vi "Sensor Simulation RT Driver VI.vi"(7 "Operation":T1, 11 "Device Reference in":T2 format="%.0x") -> (0 "Error Code":i32)   [LabVIEW 2011, in "Sensor Simulation Custom Device.lvlib"]
uses:
  Sensor Simulation Custom Device.lvlib
  <vilib>/NI Veristand/Custom Device API/Custom Device Item Ref.ctl
  <vilib>/NI Veristand/Custom Device API/Hardware Interface Driver VI Operation.ctl
  TypeDefs/SensorStateVariables.ctl
  TypeDefs/4 Wire xVDT Parameters.ctl
  TypeDefs/5 Wire xVDT Parameters.ctl
  TypeDefs/Resolver Parameters.ctl
  <userlib>/_FPGA Interface Advanced Tools/FPGA Interface Base/FPGA Interface Base.lvclass
  <vilib>/NI Veristand/Custom Device API/Block Data Reference.ctl
  <vilib>/NI Veristand/Custom Device API/Data Reference.ctl
  <vilib>/NI Veristand/Custom Device API/Data Access Type.ctl
  <vilib>/NI Veristand/Custom Device API/Custom Device Channel Type.ctl
  <userlib>/_FPGA Interface Advanced Tools/FPGA Interface Wrapper/NiFPGA Write.vi
  <userlib>/_FPGA Interface Advanced Tools/FPGA Interface Wrapper/NiFPGA Write - I32.vi
  <vilib>/NI Veristand/Custom Device API/NI VeriStand - Get Channel Values by Block Data Reference.vi
  <userlib>/_FPGA Interface Advanced Tools/FPGA Interface Base/Accessors/FPGA Read Session.vi
  <vilib>/NI Veristand/Custom Device API/Global Data Refs.vi
  <vilib>/Utility/error.llb/Error Cluster From Error Code.vi
  <vilib>/NI Veristand/Custom Device API/Custom Device API.lvlib
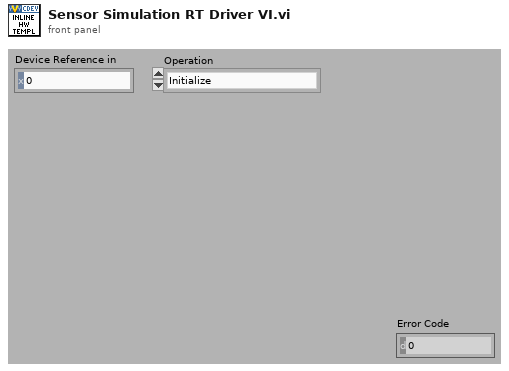
[diagram p1: front panel]
types:
  T1 = typedef "Custom Device API.lvlib/Hardware Interface Driver VI Operation.ctl" = enum16{"Initialize", "Start", "Read Data from HW", "Write Data to HW", "Close"}
  T2 = typedef "Custom Device API.lvlib/Custom Device Item Ref.ctl" = u64
  T3 = typedef "Sensor Simulation Custom Device.lvlib/SensorStateVariables.ctl" = cluster{"Device Error":errorcluster, "4 Wire xVDT Parameters ":T4[], "5 Wire xVDT Parameters":T5[], "Resolver Parameters":T6[], "FPGA Session":refnum<class "FPGA Interface Base.lvclass">, "FPGA Session Ref":u32, "Values Array":dbl[], "Block Data Refs":T7[]}
  T4 = typedef "Sensor Simulation Custom Device.lvlib/4 Wire xVDT Parameters.ctl" = cluster{"ScaleFactor1":u32, "Sensitivity":dbl, "UserDataIdx":i32, "LastUserData":dbl}
  T5 = typedef "Sensor Simulation Custom Device.lvlib/5 Wire xVDT Parameters.ctl" = cluster{"Range":dbl, "Sensitivity":dbl, "ScaleFactor1":u32, "ScaleFactor2":u32, "UserDataIdx":i32, "LastUserData":dbl}
  T6 = typedef "Sensor Simulation Custom Device.lvlib/Resolver Parameters.ctl" = cluster{"ScaleFactor1":u32, "ScaleFactor2":u32, "UserDataIdx":i32, "LastUserData":dbl}
  T7 = typedef "Custom Device API.lvlib/Block Data Reference.ctl" = cluster{"Data Reference":T8, "Offset":i32, "Length":i32}
  T8 = typedef "Custom Device API.lvlib/Data Reference.ctl" = i32
  T9 = typedef "Custom Device API.lvlib/Custom Device Channel Type.ctl" = enum16{"Input", "Output"}
  T10 = typedef "Custom Device API.lvlib/Data Access Type.ctl" = enum16{"Read", "Write"}
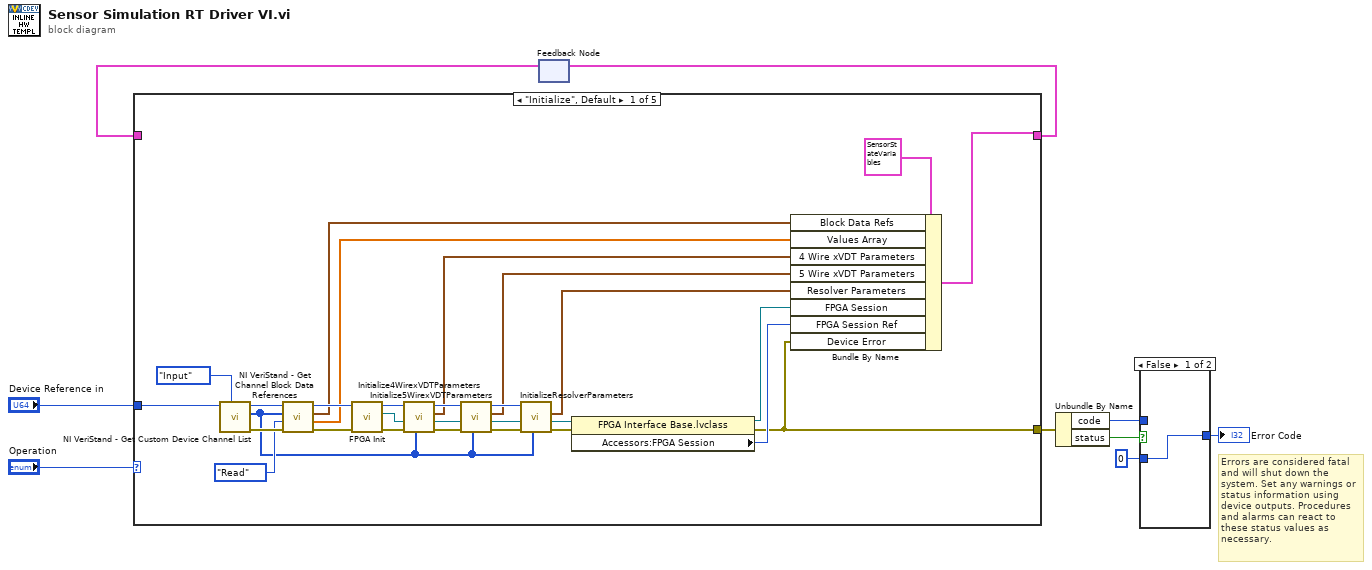
[diagram p0: block diagram]
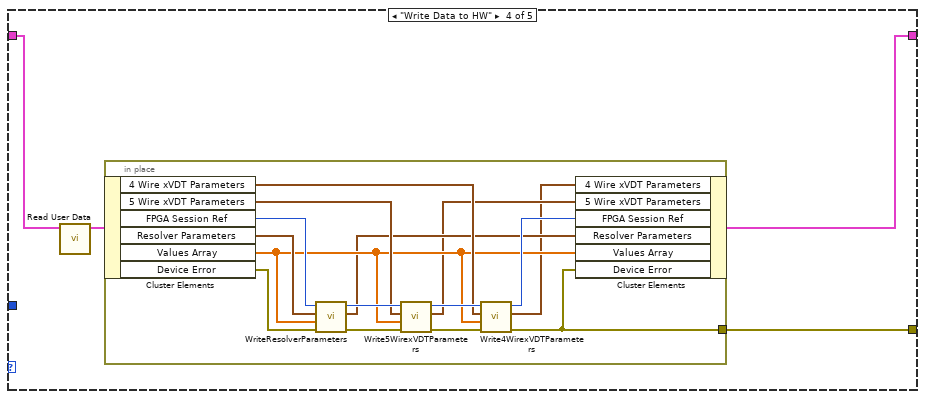
[diagram p5: hidden frame]
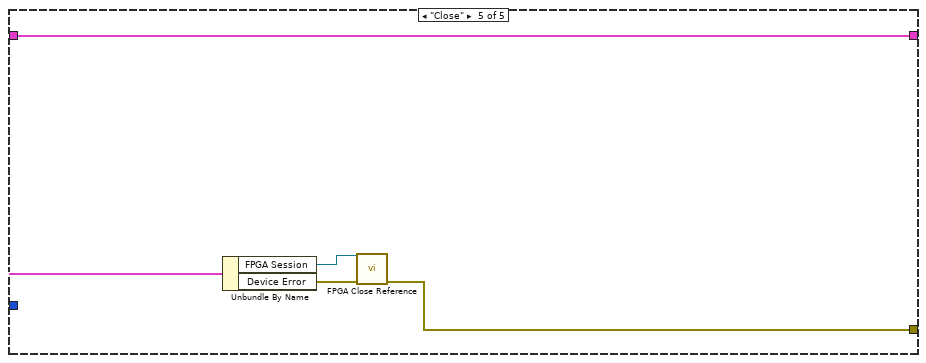
[diagram p6: hidden frame]
diagram:
  # "Errors are considered fatal and will shut down the system. Set any warnings or status information using device outputs. Procedures and alarms can react to these status values as necessary."
  n1 = feedback #1() -> (w7:T3)  [unwired: 1 out]
  n2 = case shown="\"Initialize\", Default" "Operation" {
    tunnel: [w38 w39 w40 w43 w61] -> w8
    tunnel: w7 -> [_ w39 w40 w44 w61]
    tunnel: "Device Reference in" -> [w16 _ _ _ _]
    tunnel: [w10 _ _ w41 w60] -> w5
    frame "Initialize", Default {
      n3 = call <vilib>:"NI VeriStand - Get Custom Device Channel List.vi"("Channel Type"=Custom_Device_Channel_Type."Input", "Device Ref in"=w16) -> ("error out"=w20:errorcluster, "Specified Channel Ref List"=w11:T2[], "Device Ref out"=w15:T2)  [unwired: 7 in]
      n4 = call <vilib>:"NI VeriStand - Get Channel Block Data References.vi"("error in (no error)"=w20, "Access"=Data_Access_Type."Read", "Channel Refs"=w11, "Device Ref in"=w15) -> ("error out"=w17:errorcluster, "Values Array"=w12:dbl[], "Block Data Refs"=w13:T7[], "Device Ref out"=w18:T2)  [unwired: 4 in]
      n5 = call "FPGA Init.vi"("error in (no error)"=w17, "Item Ref in"=w18) -> ("error out"=w28:errorcluster, "FPGA Session Out"=w27:refnum<class "FPGA Interface Base.lvclass">, "Item Ref Out"=w29:T2)  [unwired: 7 in]
      n6 = call "Initialize4WirexVDTParameters.vi"("Specified Channel Ref List"=w11, "error in"=w28, "FPGA Session In"=w27, "Device Reference in"=w29) -> ("error out"=w30:errorcluster, "FPGA Session Out"=w26:refnum<class "FPGA Interface Base.lvclass">, "4 Wire xVDT Parameters"=w32:T4[], "Device Reference out"=w36:T2)  [unwired: 4 in]
      n7 = call "Initialize5WirexVDTParameters.vi"("Specified Channel Ref List"=w11, "error in"=w30, "FPGA Session In"=w26, "Device Reference in"=w36) -> ("error out"=w31:errorcluster, "FPGA Session Out"=w25:refnum<class "FPGA Interface Base.lvclass">, "5 Wire xVDT Parameters"=w33:T5[], "Device Reference out"=w35:T2)  [unwired: 4 in]
      n8 = call "InitializeResolverParameters.vi"("Specified Channel Ref List"=w11, "error in"=w31, "FPGA Session In"=w25, "Device Reference in"=w35) -> ("error out"=w23:errorcluster, "FPGA Session Out"=w24:refnum<class "FPGA Interface Base.lvclass">, "Resolver Parameters"=w34:T6[])  [unwired: 4 in, 1 out]
      n9 = property class="FPGA Interface Base.lvclass"(reference=w24, error in=w23) -> (reference out=w21:refnum<class "FPGA Interface Base.lvclass">, error out=w10:errorcluster, "Accessors:FPGA Session"=w22:u32)
      n10 = Bundle By Name(cluster=T3 {"Device Error"={"status"=FALSE, "code"=0, "source"=""}, "4 Wire xVDT Parameters "=[], "5 Wire xVDT Parameters"=[], "Resolver Parameters"=[], "FPGA Session"=refnum, "FPGA Session Ref"=0, "Values Array"=[], "Block Data Refs"=[]}, "Block Data Refs"=w13, "Values Array"=w12, "4 Wire xVDT Parameters"=w32, "5 Wire xVDT Parameters"=w33, "Resolver Parameters"=w34, "FPGA Session"=w21, "FPGA Session Ref"=w22, "Device Error"=w10) -> (w38:T3)
    }
    frame "Start" {
      # "Start the device task if this action is required. This case happens after initialization before the main control loop starts running.\n\nYou can't read or write channel values in this case."
    }
    frame "Read Data from HW" {
      # "Send device output data read from HW to the system using Data References for the output channels.  Don't ever call Get or Set Channel Value by Data Reference outside the Inline Driver VI. This could cause system instability or errors."
    }
    frame "Write Data to HW" {
      n11 = call "Read User Data.vi"("RT Data in"=w44) -> ("RT Data out"=w42:T3)  [unwired: 10 in]
      n12 = in-place {
        in-place-border: [w48] -> w41
        n13 = in-place-cluster #2(w42) -> ("4 Wire xVDT Parameters"=w50:T4[], "5 Wire xVDT Parameters"=w51:T5[], "FPGA Session Ref"=w54:u32, "Resolver Parameters"=w52:T6[], "Values Array"=w49:dbl[], "Device Error"=w55:errorcluster)
        n14 = call "WriteResolverParameters.vi"("error in (no error)"=w55, "UserValues"=w49, "Resolver Parameters in"=w52, "FPGA Session"=w54) -> ("error out"=w59:errorcluster, "Resolver Parameters out"=w47:T6[], "FPGA Session Out"=w58:u32)  [unwired: 5 in]
        n15 = call "Write5WirexVDTParameters.vi"("error in (no error)"=w59, "UserValues"=w49, "5 Wire xVDT Parameters in"=w51, "FPGA Session"=w58) -> ("error out"=w56:errorcluster, "5 Wire xVDT Parameters out"=w46:T5[], "FPGA Session Out"=w57:u32)  [unwired: 5 in]
        n16 = call "Write4WirexVDTParameters.vi"("error in (no error)"=w56, "UserValues"=w49, "4 Wire xVDT Parameters  in"=w50, "FPGA Session"=w57) -> ("error out"=w48:errorcluster, "4 Wire xVDT Parameters out"=w45:T4[], "FPGA Session Out"=w53:u32)  [unwired: 5 in]
        n17 = in-place-cluster #2("4 Wire xVDT Parameters"=w45, "5 Wire xVDT Parameters"=w46, "FPGA Session Ref"=w53, "Resolver Parameters"=w47, "Values Array"=w49, "Device Error"=w48) -> (w43:T3)
      }
    }
    frame "Close" {
      n18 = Unbundle By Name(w61) -> ("FPGA Session"=w62:refnum<class "FPGA Interface Base.lvclass">, "Device Error"=w63:errorcluster)
      n19 = call-dynamic "FPGA Close Reference.vi"("error in (no error)"=w63, "FPGA Session In"=w62) -> ("error out"=w60:errorcluster)  [unwired: 9 in]
    }
  }
  n20 = feedback-in #1(w8) -> ()
  n21 = Unbundle By Name(w5) -> ("code"=w2:i32, "status"=w4:bool)
  n22 = case shown="False" w4 {
    tunnel: [w64 w65] -> w3
    tunnel: w2 -> [_ w65]
    tunnel: 0 ("f") -> [w64 _]
    frame False {
    }
    frame True {
    }
  }
  "Error Code" <- w3
